vi "DSF.Engine.Framework.Initialize Engine Buffer.vi"(8 "error in (no error)":errorcluster, 9 "channel count":u64, 10 "first channel offset":u64, 11 "Framework in":refnum<class "DSF.Engine.Framework.lvclass">) -> (0 "error out":errorcluster, 2 "Buffer":refnum<class "DSF.Engine.Pointer.DBL.lvclass">, 3 "Framework out":refnum<class "DSF.Engine.Framework.lvclass">)   [LabVIEW 2017, in "DSF.Engine.lvlib" / "DSF.Engine.Framework.lvclass"]
uses:
  DSF.Engine.Framework.lvclass
  Pointer/DSF.Engine.Pointer.DBL.lvclass
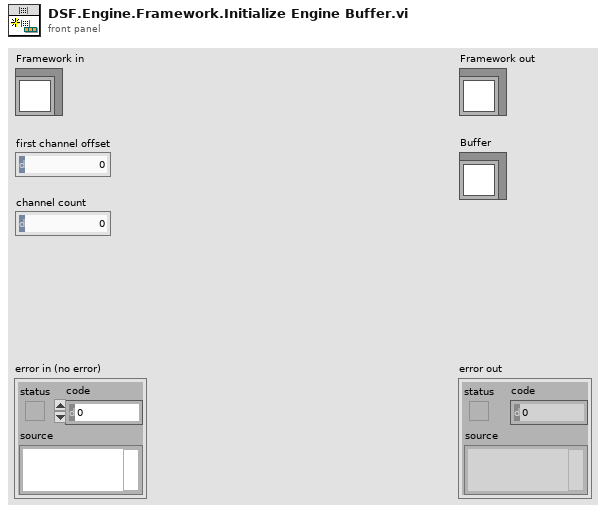
[diagram p1: front panel]
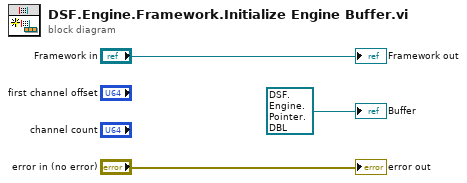
[diagram p0: block diagram]
diagram:
  "error out" <- "error in (no error)"
  "Framework out" <- "Framework in"
  "Buffer" <- refnum<class "DSF.Engine.Pointer.DBL.lvclass"> refnum ("Buffer")
